vi "loadWIPdata.vi"() -> ()   [LabVIEW 2012]
uses:
  <vilib>/addons/database/Connection.llb/DB Tools Open Connec (Path).vi
  <vilib>/addons/database/Connection.llb/Conn Execute.vi
  <vilib>/addons/database/Recordset.llb/Rec Fetch Recordset Data (R).vi
  <vilib>/addons/database/Recordset.llb/Rec Destroy - Connection.vi
  <vilib>/addons/database/_DB Variant To Data/Database Variant To Data.xnode
  <vilib>/addons/database/NI_Database_API.lvlib
panel:
  out "error out":errorcluster
  out "concatenated string":string
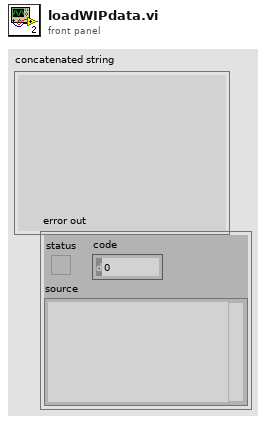
[diagram p1: front panel]
types:
  T1 = typedef "NI_Database_API.lvlib/Conn ObjectReference.ctl" = refnum<k1>
  T2 = typedef "NI_Database_API.lvlib/Rec ObjectReference.ctl" = refnum<k1>
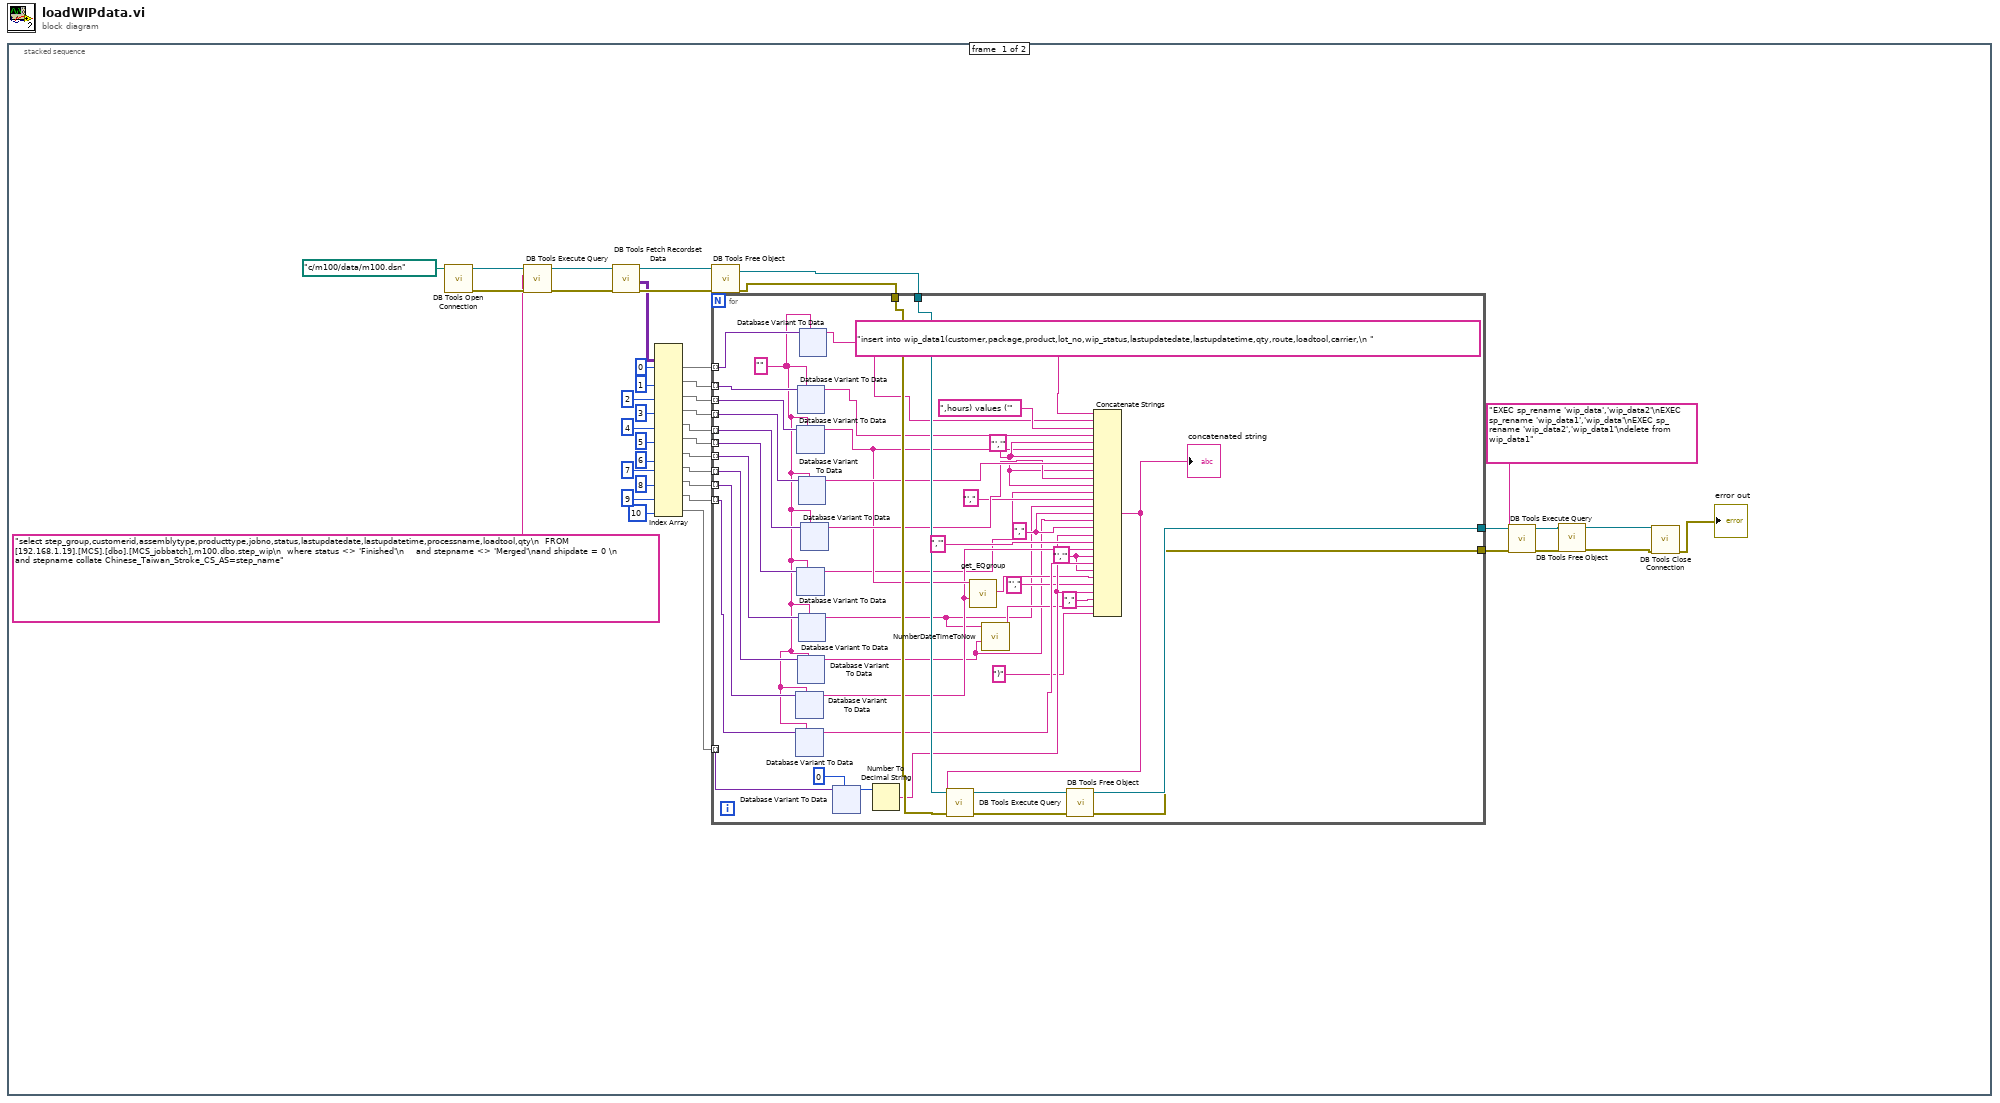
[diagram p0: block diagram]
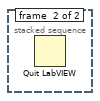
[diagram p2: hidden frame]
diagram:
  n1 = stacked-sequence {
    frame #0 {
      n2 = call-poly <vilib>:"DB Tools Open Connection.vi"("connection information"=path "c:/m100/data/m100.dsn") -> ("error out"=w38:errorcluster, "connection reference"=w41:T1)  [unwired: 7 in]
      n3 = call-poly <vilib>:"DB Tools Execute Query.vi"("error in (no error)"=w38, "SQL query"="select step_group,customerid,assemblytype,producttype,jobno,status,lastupdatedate,lastupdatetime,processname,loadtool,qty\n  FROM [192.168.1.19].[MCS].[dbo].[MCS_jobbatch],m100.dbo.step_wip\n  where status <> 'Finished'\n    and stepname <> 'Merged'\nand shipdate = 0 \n    and stepname collate Chinese_Taiwan_Stroke_CS_AS=step_name", "connection reference"=w41) -> ("error out"=w37:errorcluster, "recordset reference"=w40:T2)  [unwired: 5 in]
      n4 = call-poly <vilib>:"DB Tools Fetch Recordset Data.vi"("error in (no error)"=w37, "recordset reference"=w40) -> ("error out"=w36:errorcluster, "recordset data"=w33:variant[][], "recordset reference out"=w39:T2)  [unwired: 3 in]
      n5 = Index Array(array=w33, index (col) #1=0 ("disabled index (col)"), index (col) #2=1 ("disabled index (col)"), index (col) #3=2 ("index (col)"), index (col) #4=3 ("index (col)"), index (col) #5=4 ("index (col)"), index (col) #6=5 ("index (col)"), index (col) #7=6 ("index (col)"), index (col) #8=7 ("index (col)"), index (col) #9=8 ("index (col)"), index (col) #10=9 ("index (col)"), index (col) #11=10 ("index (col)")) -> (element #1=w14:variant[], element #2=w28:variant[], element #3=w27:variant[], element #4=w26:variant[], element #5=w25:variant[], element #6=w20:variant[], element #7=w16:variant[], element #8=w15:variant[], element #9=w4:variant[], element #10=w1:variant[], element #11=w2:variant[])  [unwired: 11 in]
      n6 = call-poly <vilib>:"DB Tools Free Object.vi"("error in (no error)"=w36, "recordset reference"=w39) -> ("error out"=w23:errorcluster, "connection reference"=w24:T1)  [unwired: 8 in]
      n7 = for {
        tunnel: w28 -> [w85] mode=indexing
        tunnel: w27 -> [w84] mode=indexing
        tunnel: w26 -> [w83] mode=indexing
        tunnel: w25 -> [w73] mode=indexing
        tunnel: w24 -> [w81]
        tunnel: w23 -> [w80]
        tunnel: [w76] -> w11
        tunnel: [w75] -> w10
        tunnel: w20 -> [w71] mode=indexing
        tunnel: w16 -> [w70] mode=indexing
        tunnel: w15 -> [w69] mode=indexing
        tunnel: w2 -> [w68] mode=indexing
        tunnel: w14 -> [w63] mode=indexing
        tunnel: w4 -> [w58] mode=indexing
        tunnel: w1 -> [w55] mode=indexing
        w48 = "','" ("string")
        w59 = "," ("string")
        w62 = "','" ("string")
        w56 = ""
        n8 = xnode "Database Variant To Data"("database variant"=w58, "type"=w56) -> ("data"=w50:string)  [unwired: 1 in, 1 out]
        n9 = xnode "Database Variant To Data"("database variant"=w55, "type"=w56) -> ("data"=w54:string)  [unwired: 1 in, 1 out]
        n10 = xnode "Database Variant To Data"("database variant"=w84, "type"=w56) -> ("data"=w51:string)  [unwired: 1 in, 1 out]
        n11 = xnode "Database Variant To Data"("database variant"=w71, "type"=w56) -> ("data"=w47:string)  [unwired: 1 in, 1 out]
        n12 = xnode "Database Variant To Data"("database variant"=w85, "type"=w56) -> ("data"=w60:string)  [unwired: 1 in, 1 out]
        n13 = xnode "Database Variant To Data"("database variant"=w69, "type"=w56) -> ("data"=w42:string)  [unwired: 1 in, 1 out]
        n14 = xnode "Database Variant To Data"("database variant"=w83, "type"=w56) -> ("data"=w74:string)  [unwired: 1 in, 1 out]
        n15 = xnode "Database Variant To Data"("database variant"=w70, "type"=w56) -> ("data"=w43:string)  [unwired: 1 in, 1 out]
        n16 = xnode "Database Variant To Data"("database variant"=w63, "type"=w56) -> ("data"=w61:string)  [unwired: 1 in, 1 out]
        n17 = xnode "Database Variant To Data"("database variant"=w73, "type"=w56) -> ("data"=w72:string)  [unwired: 1 in, 1 out]
        n18 = xnode "Database Variant To Data"("database variant"=w68, "type"=0) -> ("data"=w82:i32)  [unwired: 1 in, 1 out]
        n19 = Number To Decimal String(number=w82) -> (decimal integer string=w53:string)  [unwired: 1 in]
        n20 = call "get_EQgroup.vi"("Process"=w50, "Package"=w51) -> ("EQ Grp"=w49:string)  [unwired: 9 in]
        n21 = call "NumberDateTimeToNow.vi"("StartTime"=w42, "StartDate"=w43) -> ("Hours"=w44:string)  [unwired: 9 in]
        n22 = Concatenate Strings("insert into wip_data1(customer,package,product,lot_no,wip_status,lastupdatedate,lastupdatetime,qty,route,loadtool,carrier,\n ", w61, ",hours) values ('" ("string"), w60, w62, w51, w62, w74, w62, w72, w62, w47, "'," ("string"), w43, w59, w42, w59, w53, ",'" ("string"), w50, w48, w54, w48, w49, "'," ("string"), w53, "," ("string"), w44, ")" ("string")) -> (w77:string)
        "concatenated string" <- w77
        n23 = call-poly <vilib>:"DB Tools Execute Query.vi"("error in (no error)"=w80, "SQL query"=w77, "connection reference"=w81) -> ("error out"=w78:errorcluster, "recordset reference"=w79:T2)  [unwired: 5 in]
        n24 = call-poly <vilib>:"DB Tools Free Object.vi"("error in (no error)"=w78, "recordset reference"=w79) -> ("error out"=w75:errorcluster, "connection reference"=w76:T1)  [unwired: 8 in]
      }
      n25 = call-poly <vilib>:"DB Tools Execute Query.vi"("error in (no error)"=w10, "SQL query"="EXEC sp_rename 'wip_data','wip_data2'\nEXEC sp_rename 'wip_data1','wip_data'\nEXEC sp_rename 'wip_data2','wip_data1'\ndelete from wip_data1", "connection reference"=w11) -> ("error out"=w12:errorcluster, "recordset reference"=w9:T2)  [unwired: 5 in]
      n26 = call-poly <vilib>:"DB Tools Free Object.vi"("error in (no error)"=w12, "recordset reference"=w9) -> ("error out"=w7:errorcluster, "connection reference"=w8:T1)  [unwired: 8 in]
      n27 = call <vilib>:"DB Tools Close Connection.vi"("error in (no error)"=w7, "connection reference"=w8) -> ("error out"=→"error out":errorcluster)  [unwired: 5 in]
    }
    frame #1 {
      n28 = Quit LabVIEW() -> ()  [unwired: 1 in]
    }
  }
